vi "chart.vi"() -> ()   [LabVIEW 2016]
panel:
  out "Waveform Chart":T1(graph)
  in  "OK Button":bool
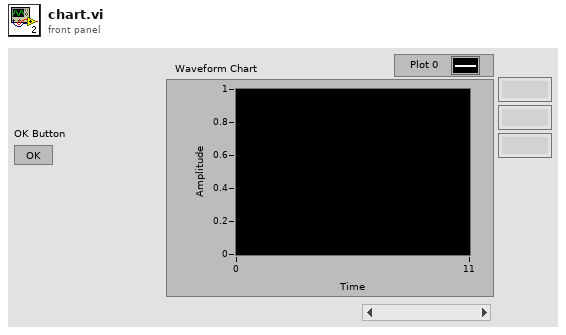
[diagram p1: front panel]
types:
  T1 = cluster{"number: 0 to 1":dbl, "number: 0 to 1":dbl, "number: 0 to 1":dbl}
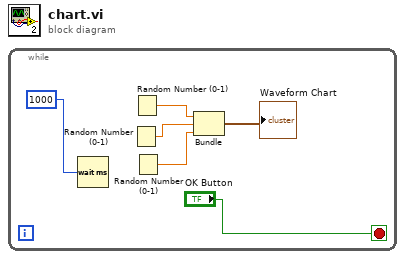
[diagram p0: block diagram]
diagram:
  n1 = while {
    stop <- "OK Button" stop-if-true
    n2 = Wait (ms)(milliseconds to wait=u32 1000) -> ()  [unwired: 1 out]
    n3 = Random Number (0-1)() -> (number: 0 to 1=w4:dbl)
    n4 = Random Number (0-1)() -> (number: 0 to 1=w5:dbl)
    n5 = Random Number (0-1)() -> (number: 0 to 1=w3:dbl)
    n6 = Bundle("number: 0 to 1"=w5, "number: 0 to 1"=w4, "number: 0 to 1"=w3) -> (→"Waveform Chart":T1)  [unwired: 1 in]
  }
